vi "test bed.vi"() -> ()   [LabVIEW 2012]
panel:
  in  "Boolean 3":bool=TRUE
  in  "Boolean 2":bool=TRUE
  in  "Boolean":bool=TRUE
  out "x < y?":bool[](array[boolean])
  out "number":u32
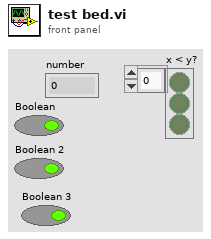
[diagram p1: front panel]
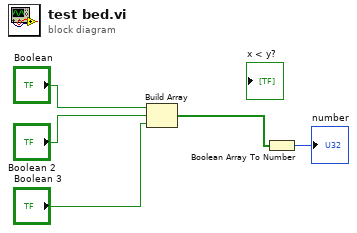
[diagram p0: block diagram]
diagram:
  n1 = Build Array("Boolean", "Boolean 2", "Boolean 3") -> (w1:bool[])
  n2 = Boolean Array To Number(Boolean array=w1) -> (number=→"number":u32)
